vi "Scan action.vi"(8 "error in (no error)":errorcluster, 9 "Indices":T1, 11 "SweepControl in":refnum<class "SweepControl.lvclass">) -> (0 "error out":errorcluster, 1 "Stop?":bool, 2 "Scan Parameters":T2={"Start"=0.14, "End"=-0.060000000000000005, "Step"=-0.060000000000000005, "Rate"=-0.060000000000000005, "wait (ms)"=10000, "address"="", "Channel"=2} {"Rate" format="%.2f"; "Step" format="%#_6p"; "End" format="%#_6p"; "Start" format="%#_6p"}, 3 "SweepControl out":refnum<class "SweepControl.lvclass">)   [LabVIEW 2016, in "SweepControl.lvclass"]
uses:
  SweepControl.lvclass
  Typedefs/Cluster - ScanParamters.ctl
  SweepControl.lvclass/SweepControl.ctl
  <userlib>/LevyLab/Levylab Instruments/Instrument.lvclass
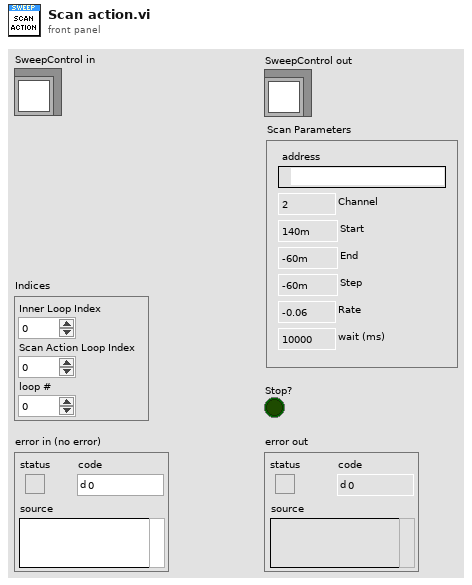
[diagram p1: front panel]
types:
  T1 = cluster{"Inner Loop Index":i32, "Scan Action Loop Index":i32, "loop #":i32}
  T2 = typedef "SweepControl.lvclass/Cluster - ScanParamters.ctl" = cluster{"Start":dbl, "End":dbl, "Step":dbl, "Rate":dbl, "wait (ms)":u32, "address":refnum<visa-resource-name>, "Channel":i32}
  T3 = typedef "SweepControl.lvclass/ScanParamters.ctl" = T2[]
  T4 = typedef "SweepControl.lvclass/ScanControl.ctl" = T5[]
  T5 = typedef "SweepControl.lvclass/Cluster - ScanControl.ctl" = cluster{"Priority":T6, "Scan name":T7}
  T6 = typedef "SweepControl.lvclass/Enum - Priority.ctl" = enum16{"Priority 0", "Priority 1", "Priority 2", "Priority 3", "Priority 4", "Priority 5"}
  T7 = typedef "SweepControl.lvclass/Enum - Action.ctl" = enum16{"OFF", "DSA_Vamp", "DSA_freq", "DSA_Vsg1", "DSA_Vsg2", "DSA_Vsg3", "DAQ_Vbg", "B_Field", "Humidity", "Temp", "MW_freq1", "MW_freq2", "MW_amplitude1", "MW_amplitude2"}
  T8 = typedef "AO-cluster.ctl" = cluster{"AO amp (V)":T9, "AO DC (V)":T10, "AO f (Hz)":T11, "AO phi (°)":T12, "function":T13, "I+":bool[]}
  T9 = typedef "AO_Amp-array.ctl" = dbl[]
  T10 = typedef "AO_DC-array.ctl" = dbl[]
  T11 = typedef "AO_f-array.ctl" = dbl[]
  T12 = typedef "AO_phi-array.ctl" = dbl[]
  T13 = typedef "Function-array.ctl" = T14[]
  T14 = typedef "Function-enum.ctl" = enum16{"Sine", "Triangle", "Square", "Sawtooth"}
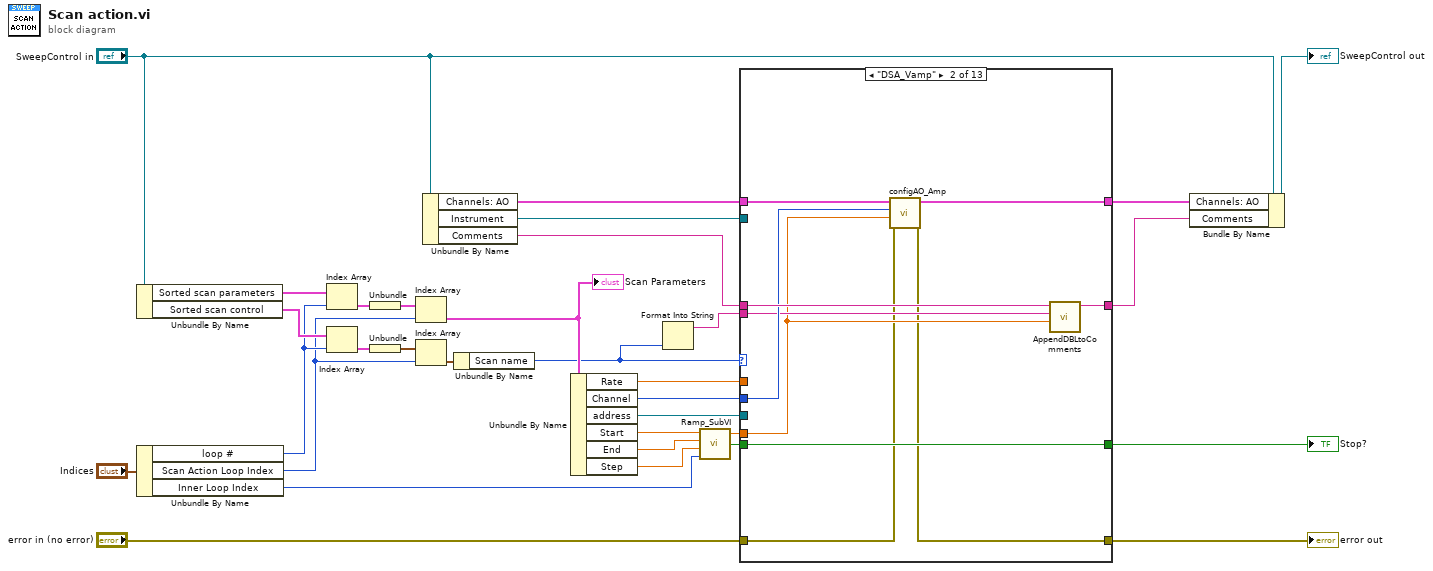
[diagram p0: block diagram]
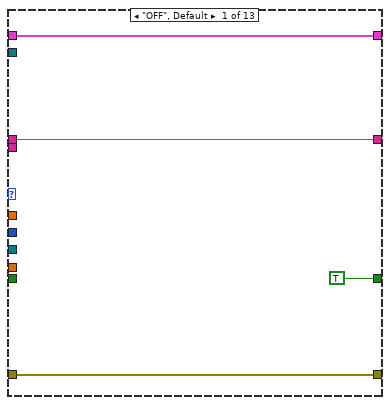
[diagram p2: hidden frame]
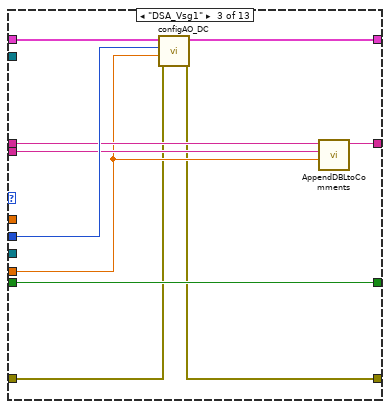
[diagram p3: hidden frame]
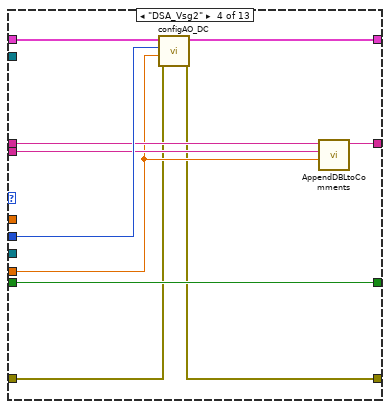
[diagram p4: hidden frame]
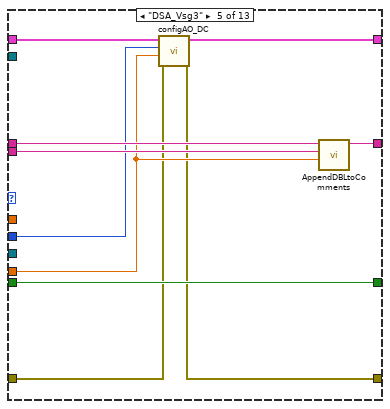
[diagram p5: hidden frame]
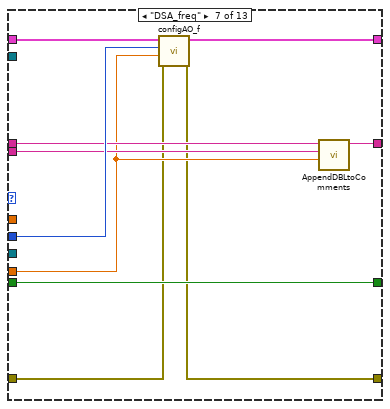
[diagram p7: hidden frame]
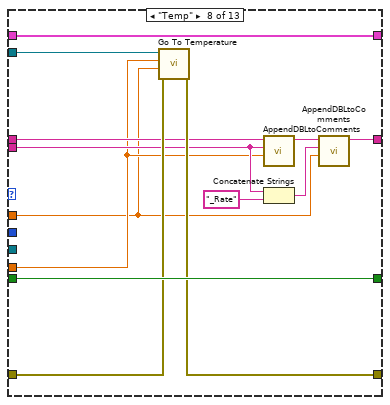
[diagram p8: hidden frame]
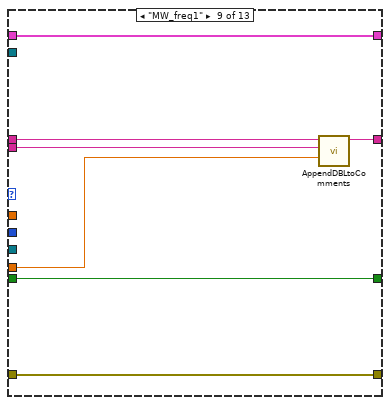
[diagram p9: hidden frame]
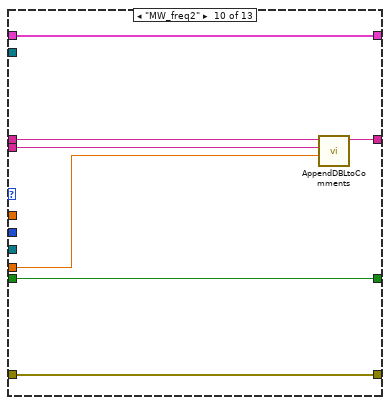
[diagram p10: hidden frame]
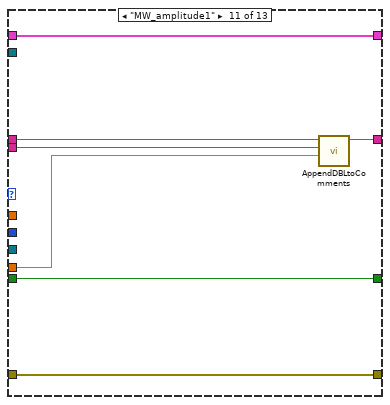
[diagram p11: hidden frame]
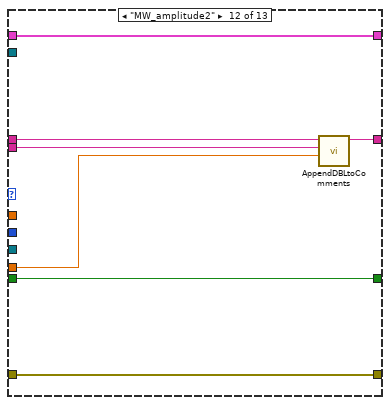
[diagram p12: hidden frame]
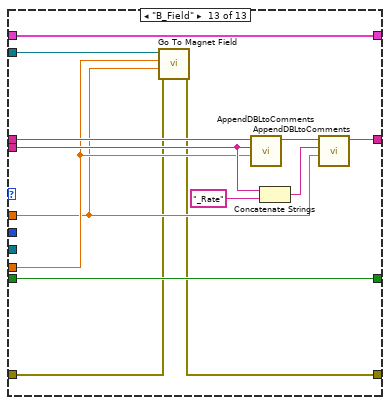
[diagram p13: hidden frame]
diagram:
  n1 = Unbundle By Name("SweepControl in") -> ("Sorted scan parameters"=w15:cluster{T3}[], "Sorted scan control"=w8:cluster{T4}[])
  n2 = Unbundle By Name("Indices") -> ("loop #"=w7:i32, "Scan Action Loop Index"=w6:i32, "Inner Loop Index"=w17:i32)
  n3 = Index Array(array=w15, index=w7) -> (element=w14:cluster{T3})
  n4 = Index Array(array=w8, index=w7) -> (element=w11:cluster{T4})
  n5 = Unbundle(w14) -> (w13:T3)
  n6 = Unbundle(w11) -> (w12:T4)
  n7 = Index Array(array=w13, index=w6) -> (element=w10:T2)
  "Scan Parameters" <- w10
  n8 = Index Array(array=w12, index=w6) -> (element=w9:T5)
  n9 = Unbundle By Name("SweepControl in") -> ("Channels: AO"=w1:T8, "Instrument"=w19:refnum<class "Instrument.lvclass">, "Comments"=w23:string)
  n10 = Unbundle By Name(w9) -> ("Scan name"=w5:T7)
  n11 = Unbundle By Name(w10) -> ("Rate"=w30:dbl, "Channel"=w32:i32, "address"=w26:refnum<visa-resource-name>, "Start"=w29:dbl, "End"=w3:dbl, "Step"=w2:dbl)
  n12 = Format Into String(w5) -> (resulting string=w4:string)  [unwired: 3 in, 1 out]
  n13 = call <userlib>:"Ramp_SubVI.vi"("index"=w17, "step"=w2, "end"=w3, "start"=w29) -> ("Stop?"=w27:bool, "Numeric"=w28:dbl)  [unwired: 1 in]
  n14 = case shown="\"DSA_Vamp\"" w5 {
    tunnel: w32 -> [_ w42 w54 w66 w69 _ w88 _ _ _ _ _ _]
    tunnel: w23 -> [w36 w46 w53 w63 w74 w79 w87 w95 w110 w116 w123 w130 w144]
    tunnel: w4 -> [_ w41 w51 w61 w72 _ w85 w94 w108 w114 w121 w128 w140]
    tunnel: [TRUE ("Stop?") w39 w49 w59 w71 w78 w83 w102 w107 w113 w120 w127 w143] -> w31
    tunnel: [w36 w45 w52 w62 w73 w79 w86 w103 w109 w115 w122 w129 w142] -> w21
    tunnel: w1 -> [w34 w44 w56 w65 w76 w80 w90 w100 w104 w117 w124 w131 w134]
    tunnel: [w34 w43 w55 w64 w75 w80 w89 w100 w104 w117 w124 w131 w134] -> w20
    tunnel: w30 -> [_ _ _ _ _ _ _ w91 _ _ _ _ w135]
    tunnel: w28 -> [_ w40 w50 w60 w70 _ w84 w92 w106 w112 w119 w126 w137]
    tunnel: w27 -> [_ w39 w49 w59 w71 w78 w83 w102 w107 w113 w120 w127 w143]
    tunnel: w26 -> [_ _ _ _ _ _ _ _ _ _ _ _ _]
    tunnel: "error in (no error)" -> [w33 w38 w48 w58 w67 w77 w82 w99 w105 w111 w118 w125 w132]
    tunnel: [w33 w37 w47 w57 w68 w77 w81 w98 w105 w111 w118 w125 w133] -> w24
    tunnel: w19 -> [_ _ _ _ _ _ _ w101 _ _ _ _ w136]
    frame "OFF", Default {
    }
    frame "DSA_Vamp" {
      n15 = call <userlib>:"configAO_Amp.vi"("error in (no error)"=w38, "new Amp (V)"=w40, "AO Channel"=w42, "Channels: AO"=w44) -> ("error out"=w37:errorcluster, "Channels: AO"=w43:T8)  [unwired: 6 in]
      n16 = call "AppendDBLtoComments.vi"("Numeric"=w40, "Label"=w41, "Comments in"=w46) -> ("Comments out"=w45:string)  [unwired: 8 in]
    }
    frame "DSA_Vsg1" {
      n17 = call <userlib>:"configAO_DC.vi"("error in (no error)"=w48, "new DC (V)"=w50, "AO Channel"=w54, "Channels: AO"=w56) -> ("error out"=w47:errorcluster, "Channels: AO"=w55:T8)  [unwired: 6 in]
      n18 = call "AppendDBLtoComments.vi"("Numeric"=w50, "Label"=w51, "Comments in"=w53) -> ("Comments out"=w52:string)  [unwired: 8 in]
    }
    frame "DSA_Vsg2" {
      n19 = call <userlib>:"configAO_DC.vi"("error in (no error)"=w58, "new DC (V)"=w60, "AO Channel"=w66, "Channels: AO"=w65) -> ("error out"=w57:errorcluster, "Channels: AO"=w64:T8)  [unwired: 6 in]
      n20 = call "AppendDBLtoComments.vi"("Numeric"=w60, "Label"=w61, "Comments in"=w63) -> ("Comments out"=w62:string)  [unwired: 8 in]
    }
    frame "DSA_Vsg3" {
      n21 = call <userlib>:"configAO_DC.vi"("error in (no error)"=w67, "new DC (V)"=w70, "AO Channel"=w69, "Channels: AO"=w76) -> ("error out"=w68:errorcluster, "Channels: AO"=w75:T8)  [unwired: 6 in]
      n22 = call "AppendDBLtoComments.vi"("Numeric"=w70, "Label"=w72, "Comments in"=w74) -> ("Comments out"=w73:string)  [unwired: 8 in]
    }
    frame "DAQ_Vbg" {
    }
    frame "DSA_freq" {
      n23 = call <userlib>:"configAO_f.vi"("error in (no error)"=w82, "new f (Hz)"=w84, "AO Channel"=w88, "Channels: AO"=w90) -> ("error out"=w81:errorcluster, "Channels: AO"=w89:T8)  [unwired: 6 in]
      n24 = call "AppendDBLtoComments.vi"("Numeric"=w84, "Label"=w85, "Comments in"=w87) -> ("Comments out"=w86:string)  [unwired: 8 in]
    }
    frame "Temp" {
      n25 = call-dynamic "Go To Temperature.vi"("error in (no error)"=w99, "Target Temperature Rate (K/min)"=w91, "Target Temperature (K)"=w92, "Instrument in"=w101) -> ("error out"=w98:errorcluster)  [unwired: 6 in, 1 out]
      n26 = call "AppendDBLtoComments.vi"("Numeric"=w92, "Label"=w94, "Comments in"=w95) -> ("Comments out"=w93:string)  [unwired: 8 in]
      n27 = Concatenate Strings(w94, "_Rate" ("string")) -> (w96:string)
      n28 = call "AppendDBLtoComments.vi"("Numeric"=w91, "Label"=w96, "Comments in"=w93) -> ("Comments out"=w103:string)  [unwired: 8 in]
    }
    frame "MW_freq1" {
      n29 = call "AppendDBLtoComments.vi"("Numeric"=w106, "Label"=w108, "Comments in"=w110) -> ("Comments out"=w109:string)  [unwired: 8 in]
    }
    frame "MW_freq2" {
      n30 = call "AppendDBLtoComments.vi"("Numeric"=w112, "Label"=w114, "Comments in"=w116) -> ("Comments out"=w115:string)  [unwired: 8 in]
    }
    frame "MW_amplitude1" {
      n31 = call "AppendDBLtoComments.vi"("Numeric"=w119, "Label"=w121, "Comments in"=w123) -> ("Comments out"=w122:string)  [unwired: 8 in]
    }
    frame "MW_amplitude2" {
      n32 = call "AppendDBLtoComments.vi"("Numeric"=w126, "Label"=w128, "Comments in"=w130) -> ("Comments out"=w129:string)  [unwired: 8 in]
    }
    frame "B_Field" {
      n33 = call-dynamic "Go To Magnet Field.vi"("error in (no error)"=w132, "Target Field Rate (T/min)"=w135, "Target Field (T)"=w137, "Instrument in"=w136) -> ("error out"=w133:errorcluster)  [unwired: 6 in, 1 out]
      n34 = call "AppendDBLtoComments.vi"("Numeric"=w137, "Label"=w140, "Comments in"=w144) -> ("Comments out"=w138:string)  [unwired: 8 in]
      n35 = Concatenate Strings(w140, "_Rate" ("string")) -> (w139:string)
      n36 = call "AppendDBLtoComments.vi"("Numeric"=w135, "Label"=w139, "Comments in"=w138) -> ("Comments out"=w142:string)  [unwired: 8 in]
    }
  }
  "Stop?" <- w31
  "error out" <- w24
  n37 = Bundle By Name(cluster="SweepControl in", "Channels: AO"=w20, "Comments"=w21) -> (→"SweepControl out":refnum<class "SweepControl.lvclass">)
